vi "Main-Strech DNA_YCC.vi"() -> ()   [LabVIEW 2014]
uses:
  <vilib>/DAQmx/create/channels.llb/DAQmx Create Channel (AI-Voltage-Basic).vi
  <vilib>/DAQmx/configure/timing.llb/DAQmx Timing (Sample Clock).vi
panel:
  out "Filtered QPD Array":dbl[][](array[numeric])
  out "Filtered Stage Array":dbl[][](array[numeric])
  out "Save to File Name Indicator":string
  out "Save to Path Indicator":path
  in  "Who's Data":enum16{"YCC", "PYW", "LCH"}(ring)
  in  "File name add to the end \n(laser power-height)":string="10mW-h300"
  in  "Save?":bool
  in  "Strech only one side?":bool=TRUE
  out "Array 3":bool[](array[boolean])
  out "Array 2":dbl[](array[numeric])
  out "Array":dbl[](array[numeric])
  out "initial position offset after move":dbl[](array[numeric])
  out "Avg. to Hz":dbl
  out "Fold QPD Signal (V)":dbl[](array[numeric])
  out "Unfold QPD Signal (V)":dbl[](array[numeric])
  out "Fold Stage Position (um)":dbl[](array[numeric])
  out "Unfold Stage Position (um)":dbl[](array[numeric])
  in  "Tab Control":T1(tab)
  out "Unfolded Graph":cluster{dbl[], dbl[]}(graph)
  out "Folded Graph":cluster{dbl[], dbl[]}(graph)
  in  "range  (um)":dbl=2.0 min=0.0 max=100.0 step=0.5 format="%.3f"
  in  "Record scan rate  (um/s)":dbl=2.0 format="%.3f"
  out "Trace direction":bool[](array[boolean])=[FALSE, TRUE, TRUE, FALSE]
  in  "Avg points":i32=200
  in  "Filter type":T2(ring)
  out "Real initial position (um)":dbl format="%0.5f"
  in  "Toward first ?\nT=+, F=-":bool
  in  "Record Mode \npath(1,2,3,4)":bool[](array[boolean])=[FALSE, FALSE, FALSE, FALSE]
  in  "Sampling rate":dbl=20000.0 format="%0.2f"
  in  "QPD value":dbl=1.0 format="%0.2f"
  in  "T=X\nF=Y":bool=TRUE
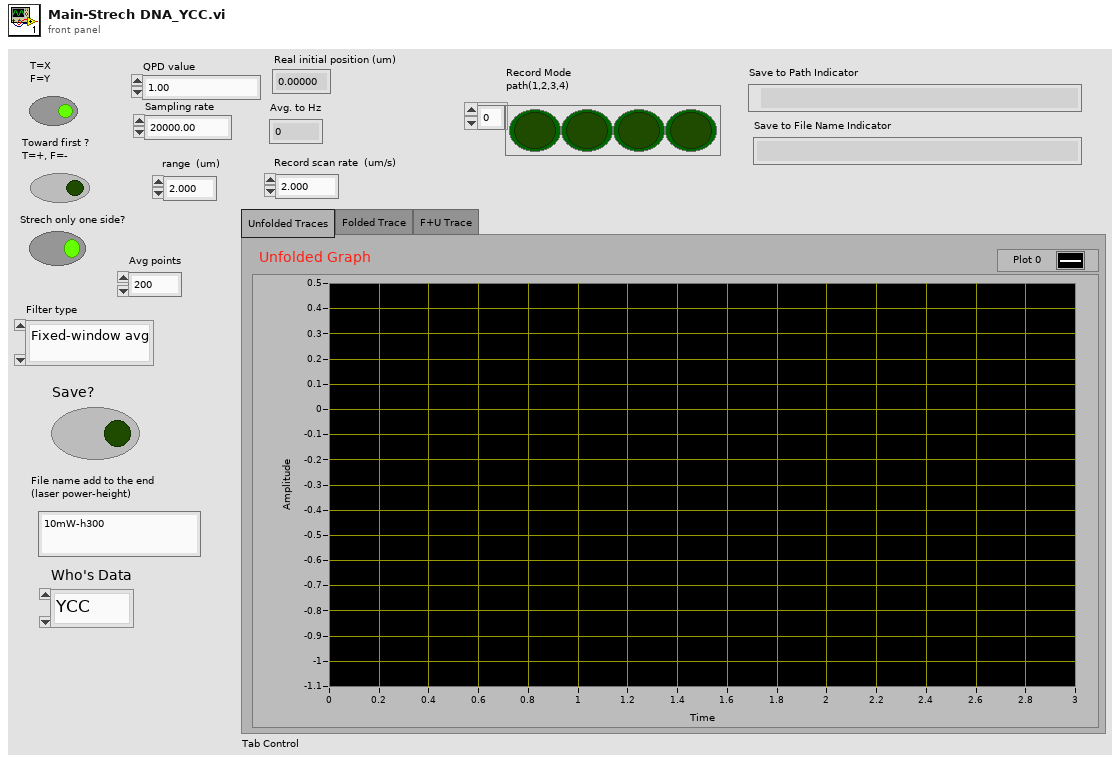
[diagram p1: front panel]
types:
  T1 = enum32{"Unfolded Traces", "Folded Trace", "F+U Trace"}
  T2 = enum16{"Fixed-window avg", "Moving-window avg", "S-G filter", "Median filter"}
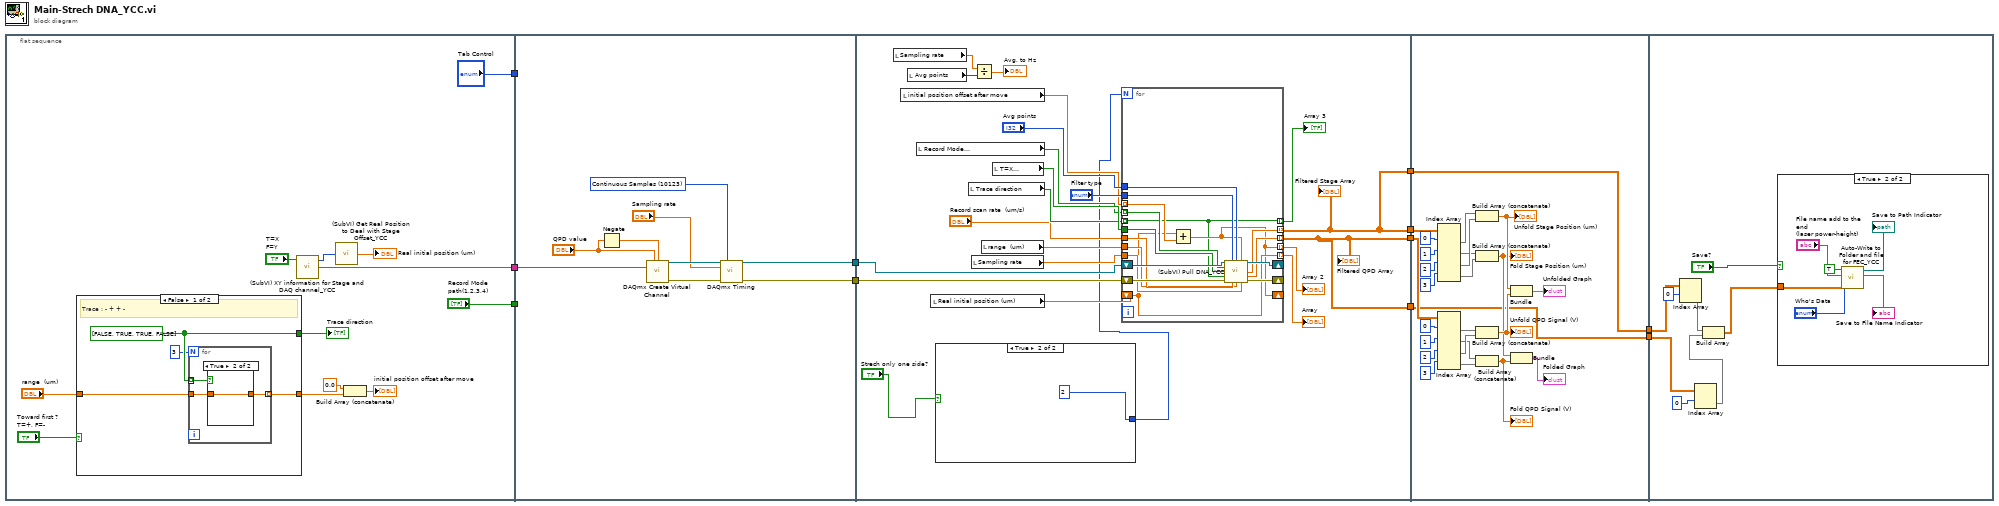
[diagram p0: block diagram]
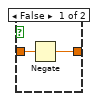
[diagram p2: hidden frame]
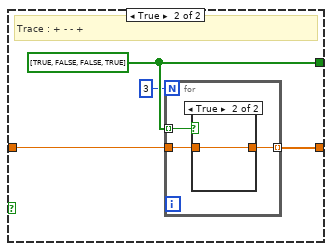
[diagram p3: hidden frame]
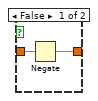
[diagram p4: hidden frame]
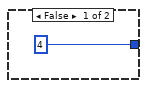
[diagram p5: hidden frame]
diagram:
  n1 = flat-sequence {
    tunnel: [w22] -> w11
    tunnel: ["Record Mode \npath(1,2,3,4)"] -> w8
    tunnel: ["Tab Control"] -> w7
    tunnel: w11 -> [w52]
    tunnel: [w45] -> w10
    tunnel: [w44] -> w9
    tunnel: w8 -> [_]
    tunnel: w7 -> [_]
    tunnel: w10 -> [w58]
    tunnel: w9 -> [w57]
    tunnel: [w54] -> w6
    tunnel: [w53] -> w5
    tunnel: [w54] -> w3
    tunnel: [w53] -> w1
    tunnel: w5 -> [w110]
    tunnel: w6 -> [w119]
    tunnel: [w95] -> w4
    tunnel: w3 -> [w95]
    tunnel: [w94] -> w2
    tunnel: w1 -> [w94]
    tunnel: w4 -> [w125]
    tunnel: w2 -> [w121]
    frame #0 {
      n2 = case shown="False" "Toward first ?\nT=+, F=-" {
        tunnel: [w27 w37] -> w18
        tunnel: "range  (um)" -> [w26 w36]
        tunnel: [w24 w35] -> w13
        frame False {
          w27 = bool[] [FALSE, TRUE, TRUE, FALSE]
          # "Trace : - + + -"
          n3 = for {
            N: 3 -> [_]
            tunnel: w27 -> [w30] mode=indexing
            tunnel: [w29] -> w24 mode=indexing
            tunnel: w26 -> [w28]
            n4 = case shown="True" w30 {
              tunnel: [w31 w33] -> w29
              tunnel: w28 -> [w32 w33]
              frame False {
                n5 = Negate(x=w32) -> (-x=w31:dbl)
              }
              frame True {
              }
            }
          }
        }
        frame True {
          w37 = bool[] [TRUE, FALSE, FALSE, TRUE]
          # "Trace : + - - +"
          n6 = for {
            N: 3 -> [_]
            tunnel: w37 -> [w40] mode=indexing
            tunnel: [w39] -> w35 mode=indexing
            tunnel: w36 -> [w38]
            n7 = case shown="True" w40 {
              tunnel: [w41 w43] -> w39
              tunnel: w38 -> [w42 w43]
              frame False {
                n8 = Negate(x=w42) -> (-x=w41:dbl)
              }
              frame True {
              }
            }
          }
        }
      }
      "Trace direction" <- w18
      n9 = call "(SubVI) XY information for Stage and DAQ channel_YCC.vi"("T=X\nF=Y"="T=X\nF=Y") -> ("physical channels"=w22:tag, "Axis"=w20:i32)  [unwired: 3 in]
      n10 = call "(SubVI) Get Real Position to Deal with Stage Offset_YCC.vi"("Axis"=w20) -> ("Real Current Commanded position (um)"=→"Real initial position (um)":dbl)  [unwired: 3 in, 1 out]
      n11 = Build Array (concatenate)(0.0, w13) -> (→"initial position offset after move":dbl[])
    }
    frame #1 {
      w47 = 10123 items=["Finite Samples"=10178, "Continuous Samples"=10123, "Hardware Timed Single Point"=12522] ("sample mode")
      n12 = Negate(x="QPD value") -> (-x=w48:dbl)
      n13 = call-poly <vilib>:"DAQmx Create Virtual Channel.vi"("maximum value"="QPD value", "minimum value"=w48, "physical channels"=w52) -> ("task out"=w50:refnum<k21>, "error out"=w51:errorcluster)  [unwired: 11 in]
      n14 = call-poly <vilib>:"DAQmx Timing.vi"("task/channels in"=w50, "sample mode"=w47, "rate"="Sampling rate", "error in"=w51) -> ("task out"=w45:refnum<k21>, "error out"=w44:errorcluster)  [unwired: 10 in]
    }
    frame #2 {
      n15 = local read "Sampling rate"() -> (w66:dbl)
      n16 = local read "initial position offset after move"() -> (w62:dbl[])
      n17 = local read "Avg points"() -> (w65:i32)
      n18 = local read "Record Mode \npath(1,2,3,4)"() -> (w68:bool[])
      n19 = local read "Real initial position (um)"() -> (w70:dbl)
      n20 = case shown="True" "Strech only one side?" {
        tunnel: [4 2] -> w55
        frame False {
        }
        frame True {
        }
      }
      n21 = local read "Trace direction"() -> (w71:bool[])
      n22 = local read "Sampling rate"() -> (w69:dbl)
      n23 = Divide(x=w66, y=w65) -> (x/y=→"Avg. to Hz":dbl)
      n24 = local read "range  (um)"() -> (w63:dbl)
      n25 = local read "T=X\nF=Y"() -> (w72:bool)
      n26 = for {
        N: w55 -> [_]
        shift-right: [w92] -> _
        shift-left: w58 -> [w93]
        shift-right: [w90] -> _
        shift-left: w57 -> [w91]
        tunnel: "Avg points" -> [w89]
        tunnel: "Filter type" -> [w88]
        tunnel: w68 -> [w87] mode=indexing
        tunnel: w72 -> [w86]
        tunnel: w71 -> [w77] mode=indexing
        tunnel: w69 -> [w85]
        tunnel: "Record scan rate  (um/s)" -> [w84]
        tunnel: w63 -> [w83]
        tunnel: [w82] -> w54 mode=indexing
        tunnel: [w81] -> w53 mode=indexing
        shift-right: [w78] -> _
        shift-left: w70 -> [w79]
        tunnel: w62 -> [w80] mode=indexing
        tunnel: [w79] -> w61 mode=indexing
        tunnel: [w78] -> w60 mode=indexing
        tunnel: [w77] -> w59 mode=indexing
        n27 = Add(x=w79, y=w80) -> (x+y=w78:dbl)
        n28 = call "(SubVI) Pull DNA_YCC.vi"("task/channels in"=w93, "Filter type"=w88, "Avg points"=w89, "Real initial position (um)"=w78, "Record?"=w87, "T=X\nF=Y"=w86, "Toward  ?\nT=+, F=-"=w77, "error in"=w91, "Record scan rate  (um/s)"=w84, "range  (um)"=w83, "Sampling rate"=w85) -> ("task out"=w92:refnum<k21>, "Filtered Stage Array"=w82:dbl[], "Filtered QPD Array"=w81:dbl[], "error out"=w90:errorcluster)  [unwired: 1 out]
      }
      "Array" <- w61
      "Array 2" <- w60
      "Array 3" <- w59
      "Filtered Stage Array" <- w54
      "Filtered QPD Array" <- w53
    }
    frame #3 {
      n29 = Index Array(array=w119, index (row) #1=0 ("index (row)"), index (row) #2=1 ("index (row)"), index (row) #3=2 ("index (row)"), index (row) #4=3 ("index (row)")) -> (element #1=w109:dbl[], element #2=w107:dbl[], element #3=w108:dbl[], element #4=w106:dbl[])  [unwired: 4 in]
      n30 = Index Array(array=w110, index (row) #1=0 ("index (row)"), index (row) #2=1 ("index (row)"), index (row) #3=2 ("index (row)"), index (row) #4=3 ("index (row)")) -> (element #1=w105:dbl[], element #2=w103:dbl[], element #3=w104:dbl[], element #4=w102:dbl[])  [unwired: 4 in]
      n31 = Build Array (concatenate)(w109, w108) -> (w101:dbl[])
      "Unfold Stage Position (um)" <- w101
      n32 = Build Array (concatenate)(w107, w106) -> (w99:dbl[])
      "Fold Stage Position (um)" <- w99
      n33 = Build Array (concatenate)(w105, w104) -> (w100:dbl[])
      "Unfold QPD Signal (V)" <- w100
      n34 = Build Array (concatenate)(w103, w102) -> (w98:dbl[])
      "Fold QPD Signal (V)" <- w98
      n35 = Bundle(w101, w100) -> (→"Unfolded Graph":cluster{dbl[], dbl[]})  [unwired: 1 in]
      n36 = Bundle(w99, w98) -> (→"Folded Graph":cluster{dbl[], dbl[]})  [unwired: 1 in]
    }
    frame #4 {
      n37 = Index Array(array=w125, index (row)=0) -> (element=w123:dbl[])  [unwired: 1 in]
      n38 = Index Array(array=w121, index (row)=0) -> (element=w120:dbl[])  [unwired: 1 in]
      n39 = Build Array(w123, w120) -> (w126:dbl[][])
      n40 = case shown="True" "Save?" {
        tunnel: w126 -> [_ w128]
        frame False {
        }
        frame True {
          n41 = call "Auto-Write to Folder and file for FEC_YCC.vi"("data to be saved"=w128, "Who's Data"="Who's Data", "File name add to the end \n(height)"="File name add to the end \n(laser power-height)", "Save?"=TRUE) -> ("Save to File Name"=→"Save to File Name Indicator":string, "Save to Path"=→"Save to Path Indicator":path)  [unwired: 4 in]
        }
      }
    }
  }
